vi "Read.vi"(7 "length":u16, 8 "error in (no error)":errorcluster, 9 "Start address":string, 10 "Read Type":variant, 11 "MelsecTCP in":refnum<class "Abs Controler.lvclass">) -> (0 "error out":errorcluster, 2 "Data":variant, 3 "MelsecTCP out":refnum<class "Abs Controler.lvclass">)   [LabVIEW 2020, in "HslCommunication.lvlib" / "Abs Controler.lvclass"]
uses:
  Abs Controler.lvclass
  E:/Git/Libraries/develop/PLCMonitor/HslCommunication/_Dependenciecs/HslCommunication.dll
  _Dependenciecs/HslCommunication.dll
  <vilib>/Utility/Data Type/NI_Data Type.lvlib
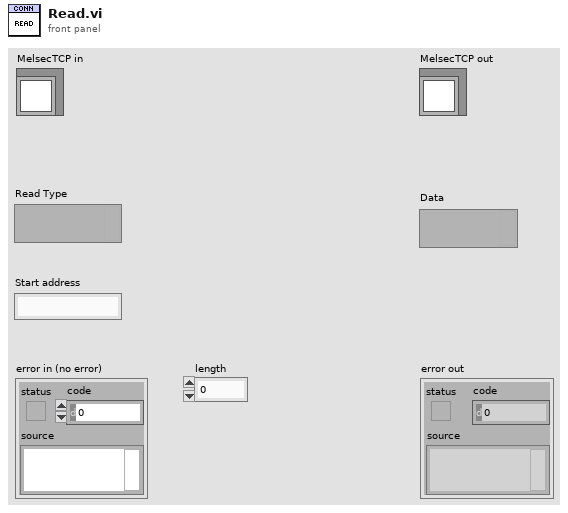
[diagram p1: front panel]
types:
  T1 = typedef "NI_Data Type.lvlib/Data Type.ctl" = enum8{"Invalid Type", "Void", "I8", "I16", "I32", "I64", "U8", "U16", "U32", "U64", "Single Float", "Double Float", "Extended Float", "Single Complex", "Double Complex", "Extended Complex", "Enum U8", "Enum U16", "Enum U32", "Enum U64", "Single Float With Unit", "Double Float With Unit", "Extended Float With Unit", "Single Complex with Unit", "Double Complex with Unit", "Extended Complex with Unit", "Boolean", "String", "Path", "Picture", "Tag", "Array", "Cluster", "Variant", "LV Variant", "Waveform", "Timestamp", "Digital Waveform", "Digital Data", "ExpressData", "Refnum", "External Data", "VI", "Poly VI", "LabVIEW Class Instance", "Fixed Point", "Set Collection", "Map Collection"}
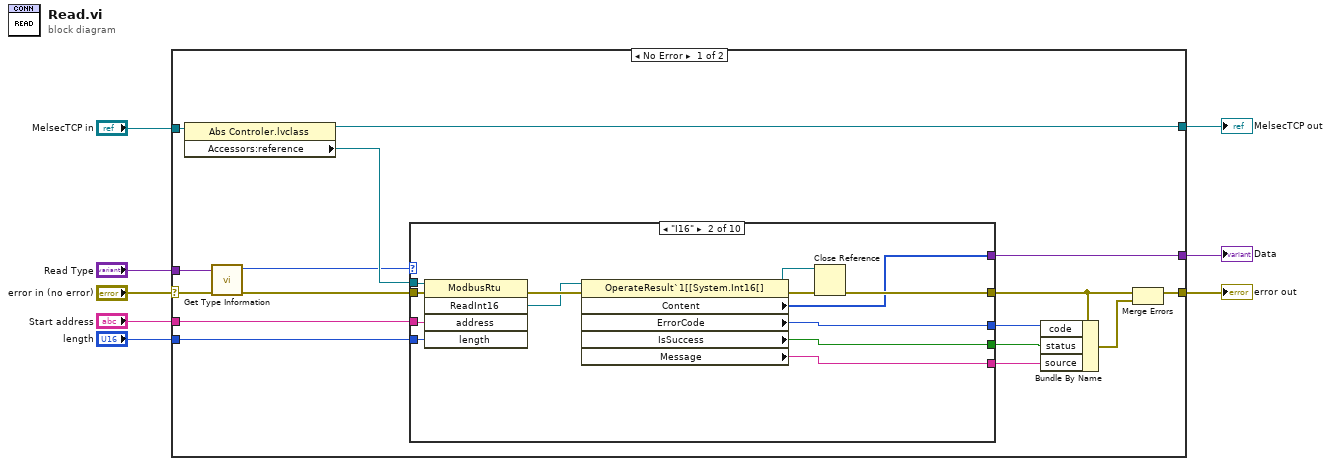
[diagram p0: block diagram]
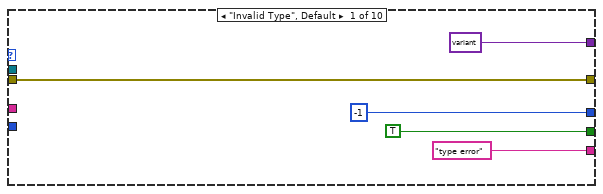
[diagram p2: hidden frame]
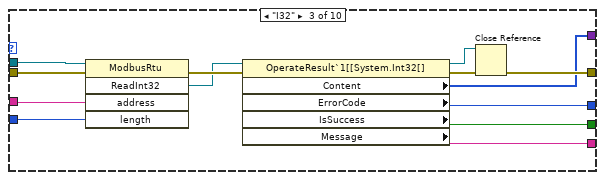
[diagram p3: hidden frame]
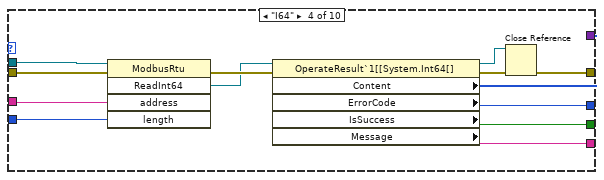
[diagram p4: hidden frame]
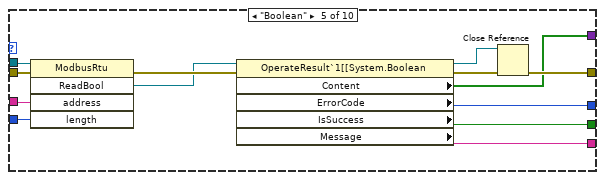
[diagram p5: hidden frame]
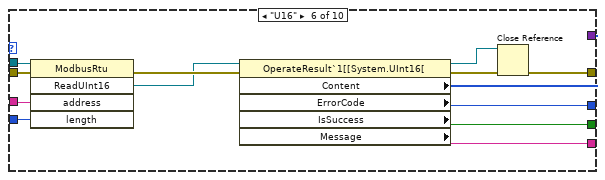
[diagram p6: hidden frame]
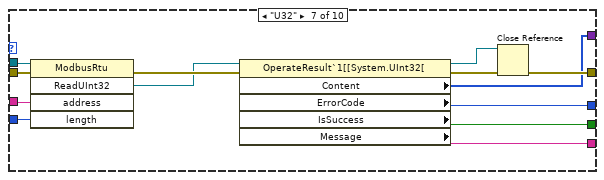
[diagram p7: hidden frame]
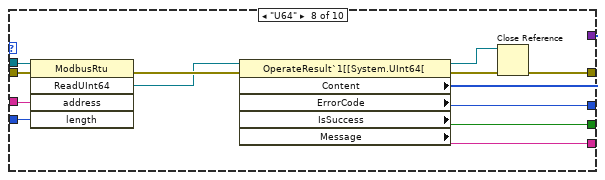
[diagram p8: hidden frame]
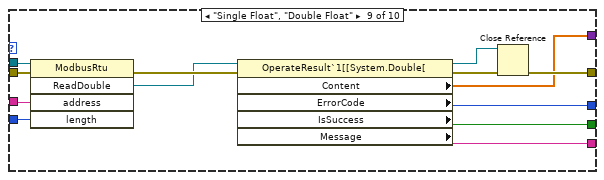
[diagram p9: hidden frame]
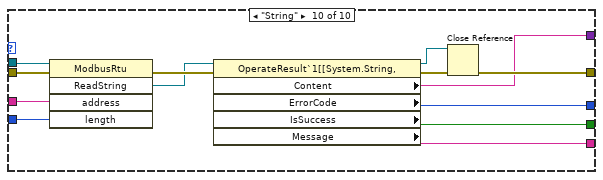
[diagram p10: hidden frame]
diagram:
  n1 = case shown="No Error" "error in (no error)" {
    selector: "error in (no error)" -> [w9 w149]
    tunnel: "MelsecTCP in" -> [w24 w148]
    tunnel: [w15 w148] -> w2
    tunnel: "Start address" -> [w12 _]
    tunnel: [w21 w149] -> w4
    tunnel: [w22 w147] -> w1
    tunnel: "length" -> [w11 _]
    tunnel: "Read Type" -> [w14 w147]
    frame No Error {
      n2 = property class="Abs Controler.lvclass"(reference=w24) -> (reference out=w15:refnum<class "Abs Controler.lvclass">, "Accessors:reference"=w23:refnum<k24>)  [unwired: 1 in, 1 out]
      n3 = call <vilib>:"Get Type Information.vi"("error in (no error)"=w9, "variant"=w14) -> ("error out"=w13:errorcluster, "type"=w10:T1)  [unwired: 5 in, 3 out]
      n4 = case shown="\"I16\"" w10 {
        tunnel: w23 -> [_ w42 w55 w68 w70 w83 w96 w109 w122 w135]
        tunnel: w12 -> [_ w41 w54 w67 w81 w94 w107 w120 w133 w146]
        tunnel: w11 -> [_ w40 w53 w66 w80 w93 w106 w119 w132 w145]
        tunnel: w13 -> [w29 w39 w52 w65 w79 w92 w105 w118 w131 w144]
        tunnel: [w29 w34 w47 w60 w74 w87 w100 w113 w126 w139] -> w17
        tunnel: [variant ("Read Type") w30 w43 w56 w69 w82 w95 w108 w121 w134] -> w22
        tunnel: [-1 ("ErrorCode") w33 w46 w59 w73 w86 w99 w112 w125 w138] -> w20
        tunnel: [TRUE ("IsSuccess") w32 w45 w58 w72 w85 w98 w111 w124 w137] -> w19
        tunnel: ["type error" ("Message") w31 w44 w57 w71 w84 w97 w110 w123 w136] -> w18
        frame "Invalid Type", Default {
        }
        frame "I16" {
          n5 = invoke class="ModbusRtu" method="ReadInt16"(reference=w42, error in=w39, "address"=w41, "length"=w40) -> (error out=w38:errorcluster, "ReadInt16"=w36:refnum<k24>)  [unwired: 1 in, 3 out]
          n6 = property class="OperateResult`1[[System.Int16[]"(reference=w36, error in=w38) -> (reference out=w35:refnum<k24>, error out=w37:errorcluster, "Content"=w30:i16[], "ErrorCode"=w33:i32, "IsSuccess"=w32:bool, "Message"=w31:string)
          n7 = Close Reference(reference=w35, error in (no error)=w37) -> (error out=w34:errorcluster)
        }
        frame "I32" {
          n8 = invoke class="ModbusRtu" method="ReadInt32"(reference=w55, error in=w52, "address"=w54, "length"=w53) -> (error out=w51:errorcluster, "ReadInt32"=w49:refnum<k24>)  [unwired: 1 in, 3 out]
          n9 = property class="OperateResult`1[[System.Int32[]"(reference=w49, error in=w51) -> (reference out=w48:refnum<k24>, error out=w50:errorcluster, "Content"=w43:i32[], "ErrorCode"=w46:i32, "IsSuccess"=w45:bool, "Message"=w44:string)
          n10 = Close Reference(reference=w48, error in (no error)=w50) -> (error out=w47:errorcluster)
        }
        frame "I64" {
          n11 = invoke class="ModbusRtu" method="ReadInt64"(reference=w68, error in=w65, "address"=w67, "length"=w66) -> (error out=w64:errorcluster, "ReadInt64"=w62:refnum<k24>)  [unwired: 1 in, 3 out]
          n12 = property class="OperateResult`1[[System.Int64[]"(reference=w62, error in=w64) -> (reference out=w61:refnum<k24>, error out=w63:errorcluster, "Content"=w56:i64[], "ErrorCode"=w59:i32, "IsSuccess"=w58:bool, "Message"=w57:string)
          n13 = Close Reference(reference=w61, error in (no error)=w63) -> (error out=w60:errorcluster)
        }
        frame "Boolean" {
          n14 = invoke class="ModbusRtu" method="ReadBool"(reference=w70, error in=w79, "address"=w81, "length"=w80) -> (error out=w78:errorcluster, "ReadBool"=w76:refnum<k24>)  [unwired: 1 in, 3 out]
          n15 = property class="OperateResult`1[[System.Boolean"(reference=w76, error in=w78) -> (reference out=w75:refnum<k24>, error out=w77:errorcluster, "Content"=w69:bool[], "ErrorCode"=w73:i32, "IsSuccess"=w72:bool, "Message"=w71:string)
          n16 = Close Reference(reference=w75, error in (no error)=w77) -> (error out=w74:errorcluster)
        }
        frame "U16" {
          n17 = invoke class="ModbusRtu" method="ReadUInt16"(reference=w83, error in=w92, "address"=w94, "length"=w93) -> (error out=w91:errorcluster, "ReadUInt16"=w89:refnum<k24>)  [unwired: 1 in, 3 out]
          n18 = property class="OperateResult`1[[System.UInt16["(reference=w89, error in=w91) -> (reference out=w88:refnum<k24>, error out=w90:errorcluster, "Content"=w82:u16[], "ErrorCode"=w86:i32, "IsSuccess"=w85:bool, "Message"=w84:string)
          n19 = Close Reference(reference=w88, error in (no error)=w90) -> (error out=w87:errorcluster)
        }
        frame "U32" {
          n20 = invoke class="ModbusRtu" method="ReadUInt32"(reference=w96, error in=w105, "address"=w107, "length"=w106) -> (error out=w104:errorcluster, "ReadUInt32"=w102:refnum<k24>)  [unwired: 1 in, 3 out]
          n21 = property class="OperateResult`1[[System.UInt32["(reference=w102, error in=w104) -> (reference out=w101:refnum<k24>, error out=w103:errorcluster, "Content"=w95:u32[], "ErrorCode"=w99:i32, "IsSuccess"=w98:bool, "Message"=w97:string)
          n22 = Close Reference(reference=w101, error in (no error)=w103) -> (error out=w100:errorcluster)
        }
        frame "U64" {
          n23 = invoke class="ModbusRtu" method="ReadUInt64"(reference=w109, error in=w118, "address"=w120, "length"=w119) -> (error out=w117:errorcluster, "ReadUInt64"=w115:refnum<k24>)  [unwired: 1 in, 3 out]
          n24 = property class="OperateResult`1[[System.UInt64["(reference=w115, error in=w117) -> (reference out=w114:refnum<k24>, error out=w116:errorcluster, "Content"=w108:u64[], "ErrorCode"=w112:i32, "IsSuccess"=w111:bool, "Message"=w110:string)
          n25 = Close Reference(reference=w114, error in (no error)=w116) -> (error out=w113:errorcluster)
        }
        frame "Single Float", "Double Float" {
          n26 = invoke class="ModbusRtu" method="ReadDouble"(reference=w122, error in=w131, "address"=w133, "length"=w132) -> (error out=w130:errorcluster, "ReadDouble"=w128:refnum<k24>)  [unwired: 1 in, 3 out]
          n27 = property class="OperateResult`1[[System.Double["(reference=w128, error in=w130) -> (reference out=w127:refnum<k24>, error out=w129:errorcluster, "Content"=w121:dbl[], "ErrorCode"=w125:i32, "IsSuccess"=w124:bool, "Message"=w123:string)
          n28 = Close Reference(reference=w127, error in (no error)=w129) -> (error out=w126:errorcluster)
        }
        frame "String" {
          n29 = invoke class="ModbusRtu" method="ReadString"(reference=w135, error in=w144, "address"=w146, "length"=w145) -> (error out=w143:errorcluster, "ReadString"=w141:refnum<k24>)  [unwired: 1 in, 3 out]
          n30 = property class="OperateResult`1[[System.String,"(reference=w141, error in=w143) -> (reference out=w140:refnum<k24>, error out=w142:errorcluster, "Content"=w134:string, "ErrorCode"=w138:i32, "IsSuccess"=w137:bool, "Message"=w136:string)
          n31 = Close Reference(reference=w140, error in (no error)=w142) -> (error out=w139:errorcluster)
        }
      }
      n32 = Bundle By Name(cluster=w17, "code"=w20, "status"=w19, "source"=w18) -> (w16:errorcluster)
      n33 = Merge Errors(w17, w16) -> (w21:errorcluster)
    }
    frame Error {
    }
  }
  "error out" <- w4
  "MelsecTCP out" <- w2
  "Data" <- w1
